vi "EndpointRead.vi"(0 "channel in":T1, 1 "timeout in ms (-1)":i32=-1, 12 "abort (F)":bool) -> (3 "timed out?":bool, 6 "valid?":bool, 8 "element out":T2, 13 "count":i32, 14 "aborted?":bool, 15 "last element?":bool)   [LabVIEW 2017, in "Stream-t'WPI_EncoderType.ctl'.lvlib"]
uses:
  <extravilib>/ChannelInstances/Stream-t'WPI_EncoderType.ctl'.lvlib
  <vilib>/Rock Robotics/WPI/Encoder/WPI_EncoderType.ctl
  <extravilib>/ChannelInstances/Stream-t'WPI_EncoderType.ctl'/)Channel.ctl
  <extravilib>/ChannelInstances/Stream-t'WPI_EncoderType.ctl'/ChannelOp.ctl
  <resource>/ChannelSupport/_ChannelSupport/_ChannelSupport.lvlib
panel:
  # "legal combinations:\n\n    abort\n    timedout\n    valid\n    valid, last element\n    last element"
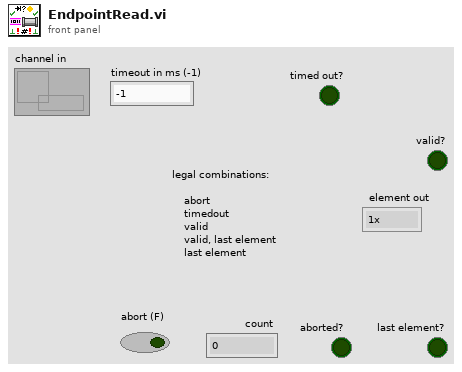
[diagram p1: front panel]
types:
  T1 = typedef "Stream-t'WPI_EncoderType.ctl'.lvlib/)Channel.ctl" = refnum<queue>
  T2 = typedef "WPI_EncoderType.ctl" = enum16{"1x", "2x", "4x"}
  T3 = typedef "Stream-t'WPI_EncoderType.ctl'.lvlib/ChannelOp.ctl" = enum16{"init", "write", "read", "probe"}
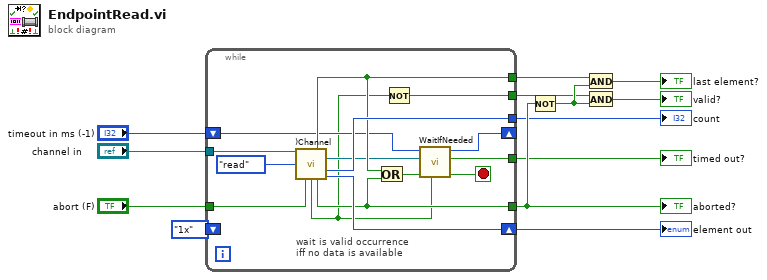
[diagram p0: block diagram]
diagram:
  n1 = while {
    tunnel: "channel in" -> [w28]
    tunnel: [w23] -> w11
    tunnel: [w20] -> w10
    tunnel: [w22] -> w4
    tunnel: [w27] -> w9
    tunnel: [w14] -> w2
    tunnel: "abort (F)" -> [w25]
    shift-right: [w17] -> _
    shift-left: "timeout in ms (-1)" -> [w19]
    shift-right: [w26] -> w6
    shift-left: WPI_EncoderType."1x" ("element out") -> [_]
    stop <- w21 stop-if-true
    # "wait is valid occurrence\niff no data is available"
    n2 = call <extravilib>:")Channel.vi"("channel in"=w28, "channelOp"=ChannelOp."read", "abort in"=w25) -> ("last element out"=w22:bool, "wait"=w16:refnum<k4>, "count"=w27:i32, "retry"=w15:bool, "aborted"=w23:bool, "element out"=w26:T2)  [unwired: 5 in, 2 out]
    n3 = Or(x=w22, y=w23) -> (x .or. y?=w18:bool)
    n4 = Not(x=w15) -> (.not. x?=w14:bool)
    n5 = call <resource>:"WaitIfNeeded.vi"("retry"=w15, "stopping"=w18, "wait"=w16, "_timeout (ms) in"=w19) -> ("stop loop"=w21:bool, "timed out"=w20:bool, "_timeout (ms) out"=w17:i32)  [unwired: 5 in]
  }
  "element out" <- w6
  "count" <- w9
  "timed out?" <- w10
  "aborted?" <- w11
  n6 = Not(x=w11) -> (.not. x?=w3:bool)
  n7 = And(x=w4, y=w3) -> (x .and. y?=→"last element?":bool)
  n8 = And(x=w2, y=w3) -> (x .and. y?=→"valid?":bool)
